vi "SP Perform Filter Bandwidth Limit Testing.vi"(6 "Limit Results In":T2={"Limit #"=0, "Parameter"={"Stimulus Port"=1, "Response Port"=0}, "Bandwidth Pass?"={"Pass?"=FALSE, "Bandwidth"=0.0, "Limit"=0.0, "Units"=enum."Hz"}, "Ripple Pass?"={"Pass?"=FALSE, "Ripple"=0.0, "Limit"=0.0, "Format"=enum."Log Mag"}, "Attenuation Results"=[], "Skirt Results"=[], "Pass?"=FALSE} {"Parameter"."Stimulus Port" min=1 step=1; "Parameter"."Response Port" min=1 step=1}, 8 "error in (no error)":errorcluster, 10 "Data":T10={"F0"=500.0, "dF"=1.0, "Formatted Values"=[-6.0, -6.0, -6.0, -6.0, -6.0, -6.0, -5.0, -4.0, -3.0, -2.0, -1.0017226002993769, -0.8636286738753696, -1.012432061728755, -0.8135188671805874, -1.084383696215112, -1.192695586219516, -0.8228939725524264, -1.1588169801015764, -1.0069715761898415, -0.8118111488159718, -0.9516999033989667, -1.0842662636672022, -1.0261931083967077, -0.816874162233468, -0.8335770068326294, -1.1794529347576463, -1.1032959879886735, -1.197742447623333, -0.9631229100196212, -0.9908453124177325, -0.9835470980893588, -1.10217991844936, -0.8956607286257672, -0.8794782872077156, -0.9013683651609963, -1.0772188731817596, -0.992723355191172, -0.9536275499498994, -0.9874327685983141, -0.921963653527827, -0.8848787728556787, -1.1874980208218, -0.996957511881206, -0.9972503730309241, -0.8866139538542095, -1.07344181331393, -0.881559772443858, -1.0112449407130875, -0.9865384477979471, -0.9901446738263366, -1.1718630063784758, -0.9951725256878827, -0.931778781153855, -0.9846289731021831, -0.851763264124267, -0.9086965469391421, -0.8349429101974368, -0.8383742350256687, -1.106571816484691, -0.9554005266395742, -0.9376822403043366, -1.131287512516927, -1.0382288806403288, -0.917054052988136, -0.9489467877812984, -0.9264227759143271, -1.0918690925892351, -1.1668737446636852, -1.0021735712381068, -1.1541225361979714, -1.1931131329605709, -0.8730502330378824, -0.850411285659811, -1.137775166801135, -1.1870586525662095, -1.0926571181161528, -1.118993526927924, -1.1211410787283602, -0.8920697041785735, -0.888430731015914, -1.0656600076605476, -1.1666787859795846, -1.0713340188424678, -0.8625910088884297, -1.1434360227216422, -0.9217710376784376, -1.1218396445954617, -0.9558195687190933, -1.1773692443654946, -1.0827782751424972, -1.1567791336122029, -0.8684407402614696, -0.8177845157195978, -0.9040657051180614, -0.9313557288389804, -1.0236831450620423, -1.050426714979035, -0.8344777069605718, -0.8274082929927138, -1.1990080831766776, -1.0947798998491134, -1.1963114865246718, -1.0016247375583676, -1.0877110100652403, -1.1556028882288836, -1.1918380581525247, -0.9751292214691399, -0.8884133044813358, -1.0347444321214612, -0.9445125246491541, -2.0, -3.0, -4.0, -5.0, -6.0, -6.0, -6.0, -6.0, -6.0, -6.0]}, 11 "Filter Limit":T11={"Limit #"=1, "Parameter"={"Stimulus Port"=1, "Response Port"=2}, "Format"=enum."Log Mag", "Filter Type"=enum."Bandpass", "Passband"={"Start/Center"=510.0, "Stop/Span"=610.0, "Units"=enum."MHz", "Freq Format"=enum."Start/Stop", "Bandwidth Attn"=3.0, "Passband Limit"=FALSE}, "Ripple"={"Ripple Limit"=TRUE, "Window On"=FALSE, "Ripple"=0.1, "Window"=10.0, "Units"=enum."MHz"}, "Attenuation Points"=[], "Skirt Points"=[]} {"Parameter"."Stimulus Port" min=1 step=1; "Parameter"."Response Port" min=1 step=1; "Passband"."Bandwidth Attn" format="%.3g"; "Passband"."Stop/Span" format="%.3g"; "Passband"."Start/Center" format="%.3g"}) -> (0 "error out":errorcluster, 2 "Results":T1, 3 "Pass?":bool, 4 "Limit Results Out":T2={"Limit #"=0, "Parameter"={"Stimulus Port"=1, "Response Port"=0}, "Bandwidth Pass?"={"Pass?"=FALSE, "Bandwidth"=0.0, "Limit"=0.0, "Units"=enum."Hz"}, "Ripple Pass?"={"Pass?"=FALSE, "Ripple"=0.0, "Limit"=0.0, "Format"=enum."Log Mag"}, "Attenuation Results"=[], "Skirt Results"=[], "Pass?"=FALSE} {"Parameter"."Stimulus Port" min=1 step=1; "Parameter"."Response Port" min=1 step=1})   [LabVIEW 2011]
uses:
  TypeDefs/SP Filter.ctl
  TypeDefs/SP Parameter.ctl
  TypeDefs/SP Format.ctl
  TypeDefs/SP Filter Type.ctl
  TypeDefs/SP Filter Passband.ctl
  TypeDefs/SP Frequency Units.ctl
  TypeDefs/SP Frequency Format.ctl
  TypeDefs/SP Filter Ripple.ctl
  TypeDefs/SP Attenuation Point.ctl
  TypeDefs/SP Attenuation Type.ctl
  TypeDefs/SP Skirt Rejection Point.ctl
  TypeDefs/SP Relative Loss.ctl
  TypeDefs/SP Limit Results.ctl
  TypeDefs/SP Bandwidth Limit Results.ctl
  TypeDefs/SP Ripple Limit Results.ctl
  TypeDefs/SP Attenuation Limit Results.ctl
  TypeDefs/SP Skirt Limit Results.ctl
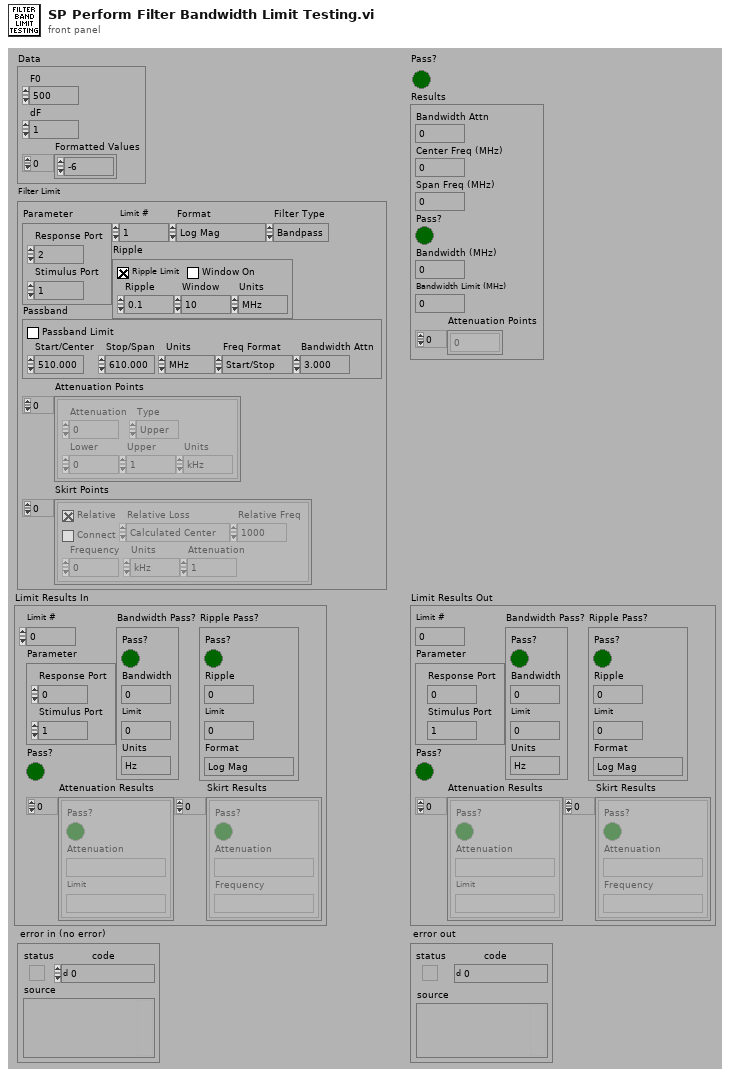
[diagram p1: front panel]
types:
  T1 = cluster{"Bandwidth Attn":dbl, "Center Freq (MHz)":dbl, "Span Freq (MHz)":dbl, "Pass?":bool, "Bandwidth (MHz)":dbl, "Bandwidth Limit (MHz)":dbl, "Attenuation Points":dbl[]}
  T2 = typedef "SP Limit Results.ctl" = cluster{"Limit #":i8, "Parameter":T3, "Bandwidth Pass?":T4, "Ripple Pass?":T6, "Attenuation Results":T8[], "Skirt Results":T9[], "Pass?":bool}
  T3 = typedef "SP Parameter.ctl" = cluster{"Stimulus Port":i8, "Response Port":i8}
  T4 = typedef "SP Bandwidth Limit Results.ctl" = cluster{"Pass?":bool, "Bandwidth":dbl, "Limit":dbl, "Units":T5}
  T5 = typedef "SP Frequency Units.ctl" = enum16{"Hz", "kHz", "MHz", "GHz", "Points"}
  T6 = typedef "SP Ripple Limit Results.ctl" = cluster{"Pass?":bool, "Ripple":dbl, "Limit":dbl, "Format":T7}
  T7 = typedef "SP Format.ctl" = enum16{"Log Mag", "Lin Mag", "SWR", "Phase", "Expanded Phase", "Delay", "Insertion Loss", "Isolation", "Return Loss"}
  T8 = typedef "SP Attenuation Limit Results.ctl" = cluster{"Pass?":bool, "Attenuation":string, "Limit":string}
  T9 = typedef "SP Skirt Limit Results.ctl" = cluster{"Pass?":bool, "Attenuation":string, "Frequency":string}
  T10 = cluster{"F0":dbl, "dF":dbl, "Formatted Values":dbl[]}
  T11 = typedef "SP Filter.ctl" = cluster{"Limit #":i8, "Parameter":T3, "Format":T7, "Filter Type":T12, "Passband":T13, "Ripple":T15, "Attenuation Points":T16[], "Skirt Points":T18[]}
  T12 = typedef "SP Filter Type.ctl" = enum16{"Lowpass", "Highpass", "Bandpass", "Bandstop"}
  T13 = typedef "SP Filter Passband.ctl" = cluster{"Start/Center":dbl, "Stop/Span":dbl, "Units":T5, "Freq Format":T14, "Bandwidth Attn":dbl, "Passband Limit":bool}
  T14 = typedef "SP Frequency Format.ctl" = enum16{"Start/Stop", "Center/Span"}
  T15 = typedef "SP Filter Ripple.ctl" = cluster{"Ripple Limit":bool, "Window On":bool, "Ripple":dbl, "Window":dbl, "Units":T5}
  T16 = typedef "SP Attenuation Point.ctl" = cluster{"Attenuation":dbl, "Type":T17, "Lower":dbl, "Upper":dbl, "Units":T5}
  T17 = typedef "SP Attenuation Type.ctl" = enum16{"Center", "Lower", "Upper"}
  T18 = typedef "SP Skirt Rejection Point.ctl" = cluster{"Relative":bool, "Connect":bool, "Frequency":dbl, "Units":T5, "Attenuation":dbl, "Relative Loss":T19, "Relative Freq":dbl}
  T19 = typedef "SP Relative Loss.ctl" = enum16{"Calculated Center", "Passband Minimum", "Passband Maximum", "Passband Average", "Frequency"}
  T20 = cluster{"Bandwidth Attn":dbl, "Start/Center Out":dbl, "Stop/Span Out":dbl, bool, "Interpolated X Value":dbl, "Stop/Span Out":dbl, dbl[]}
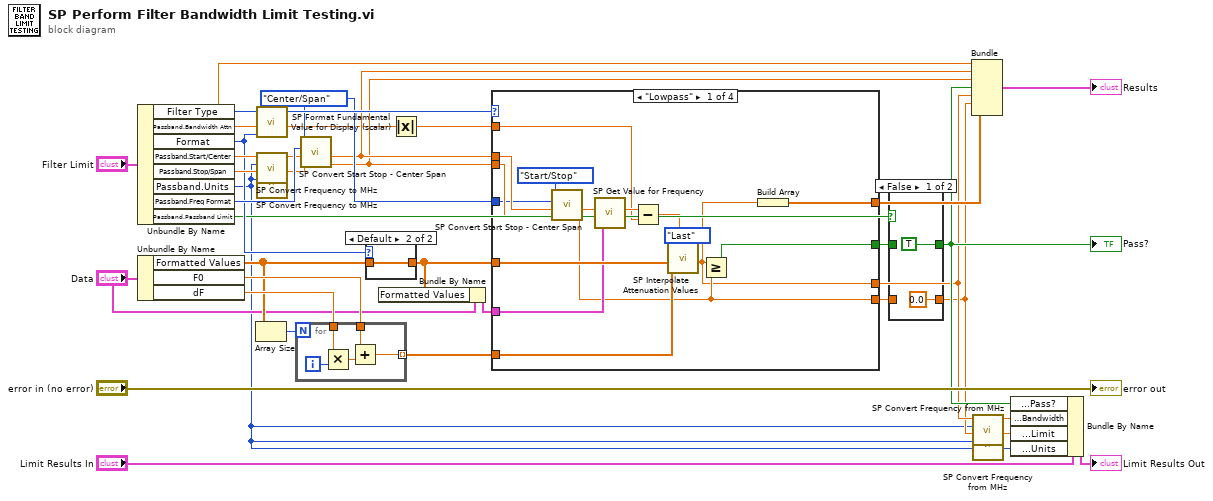
[diagram p0: block diagram]
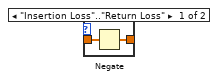
[diagram p3: hidden frame]
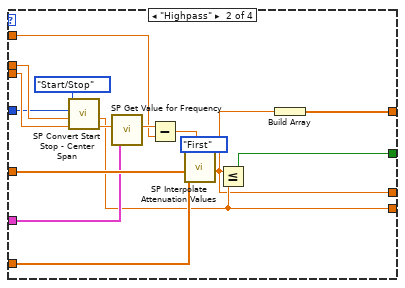
[diagram p4: hidden frame]
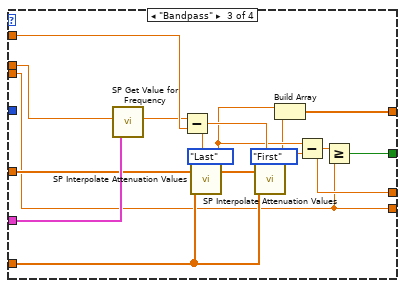
[diagram p5: hidden frame]
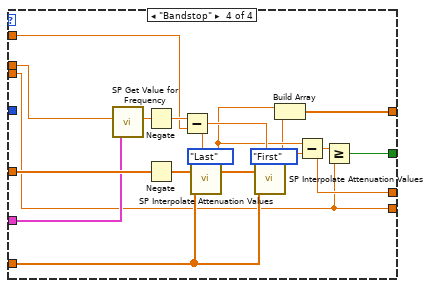
[diagram p6: hidden frame]
diagram:
  w17 = SP_Frequency_Format."Center/Span" ("Freq Format To")
  n1 = Unbundle By Name("Filter Limit") -> ("Filter Type"=w35:T12, "Passband.Bandwidth Attn"=w25:dbl, "Format"=w24:T7, "Passband.Start/Center"=w34:dbl, "Passband.Stop/Span"=w33:dbl, "Passband.Units"=w1:T5, "Passband.Freq Format"=w27:T14, "Passband.Passband Limit"=w9:bool)
  n2 = Unbundle By Name("Data") -> ("Formatted Values"=w23:dbl[], "F0"=w32:dbl, "dF"=w31:dbl)
  n3 = Array Size(array=w23) -> (size(s)=w21:i32)
  n4 = call "SP Format Fundamental Value for Display (scalar).vi"("Format"=w24, "Stored Value (0, linear)"=w25) -> ("Display Value"=w14:dbl)  [unwired: 5 out]
  n5 = call "SP Convert Frequency to MHz.vi"("Units"=w1, "Frequency"=w34) -> ("Converted Frequency"=w19:dbl)  [unwired: 1 in, 8 out]
  n6 = call "SP Convert Frequency to MHz.vi"("Units"=w1, "Frequency"=w33) -> ("Converted Frequency"=w18:dbl)  [unwired: 1 in, 8 out]
  n7 = for {
    N: w21 -> [_]
    tunnel: w31 -> [w40]
    tunnel: w32 -> [w38]
    tunnel: [w37] -> w20 mode=indexing
    i -> [w41]
    n8 = Multiply(x=w40, y=w41) -> (x*y=w39:dbl)
    n9 = Add(x=w38, y=w39) -> (x+y=w37:dbl)
  }
  n10 = call "SP Convert Start Stop - Center Span.vi"("Stop/Span In"=w18, "Start/Center In"=w19, "Freq Format From"=w27, "Freq Format To"=w17) -> ("Stop/Span Out"=w15:dbl, "Start/Center Out"=w16:dbl)  [unwired: 6 out]
  n11 = case shown="Default" w24 {
    tunnel: w23 -> [w43 w44]
    tunnel: [w42 w44] -> w11
    frame "Insertion Loss".."Return Loss" {
      n12 = Negate(x=w43) -> (-x=w42:dbl[])
    }
    frame Default {
    }
  }
  n13 = Bundle By Name(cluster="Data", "Formatted Values"=w11) -> (w12:T10)
  n14 = Absolute Value(x=w14) -> (abs(x)=w13:dbl)
  n15 = case shown="\"Lowpass\"" w35 {
    tunnel: w16 -> [w56 w72 w81 w95]
    tunnel: w15 -> [w55 w71 w80 w96]
    tunnel: w17 -> [w54 w70 _ _]
    tunnel: w11 -> [w59 w75 w84 w102]
    tunnel: w13 -> [w51 w67 w86 w99]
    tunnel: w20 -> [w58 w74 w88 w101]
    tunnel: w12 -> [w53 w69 w87 w100]
    tunnel: [w49 w65 w85 w98] -> w8
    tunnel: [w46 w61 w82 w97] -> w5
    tunnel: [w47 w63 w80 w96] -> w7
    tunnel: [w45 w62 w77 w92] -> w10
    frame "Lowpass" {
      n16 = call "SP Convert Start Stop - Center Span.vi"("Stop/Span In"=w55, "Start/Center In"=w56, "Freq Format From"=w54, "Freq Format To"=SP_Frequency_Format."Start/Stop") -> ("Stop/Span Out"=w47:dbl, "Start/Center Out"=w48:dbl)  [unwired: 6 out]
      n17 = call "SP Get Value for Frequency.vi"("Data"=w53, "Frequency (MHz)"=w48) -> ("Value"=w52:dbl)  [unwired: 5 out]
      n18 = Subtract(x=w52, y=w51) -> (x-y=w50:dbl)
      n19 = call "SP Interpolate Attenuation Values.vi"("Instance (First)"=enum16{"First", "Last"}."Last", "Attenuation Value"=w50, "X Values"=w58, "Y Values"=w59) -> ("Interpolated X Value"=w46:dbl)  [unwired: 7 out]
      n20 = Greater Or Equal?(x=w46, y=w47) -> (x >= y?=w49:bool)
      n21 = Build Array(w46) -> (w45:dbl[])
    }
    frame "Highpass" {
      n22 = call "SP Convert Start Stop - Center Span.vi"("Stop/Span In"=w71, "Start/Center In"=w72, "Freq Format From"=w70, "Freq Format To"=SP_Frequency_Format."Start/Stop") -> ("Stop/Span Out"=w64:dbl, "Start/Center Out"=w63:dbl)  [unwired: 6 out]
      n23 = call "SP Get Value for Frequency.vi"("Data"=w69, "Frequency (MHz)"=w64) -> ("Value"=w68:dbl)  [unwired: 5 out]
      n24 = Subtract(x=w68, y=w67) -> (x-y=w66:dbl)
      n25 = call "SP Interpolate Attenuation Values.vi"("Instance (First)"=enum16{"First", "Last"}."First", "Attenuation Value"=w66, "X Values"=w74, "Y Values"=w75) -> ("Interpolated X Value"=w61:dbl)  [unwired: 7 out]
      n26 = Less Or Equal?(x=w61, y=w63) -> (x <= y?=w65:bool)
      n27 = Build Array(w61) -> (w62:dbl[])
    }
    frame "Bandpass" {
      n28 = call "SP Get Value for Frequency.vi"("Data"=w87, "Frequency (MHz)"=w81) -> ("Value"=w83:dbl)  [unwired: 5 out]
      n29 = Subtract(x=w83, y=w86) -> (x-y=w89:dbl)
      n30 = call "SP Interpolate Attenuation Values.vi"("Instance (First)"=enum16{"First", "Last"}."Last", "Attenuation Value"=w89, "X Values"=w88, "Y Values"=w84) -> ("Interpolated X Value"=w79:dbl)  [unwired: 7 out]
      n31 = call "SP Interpolate Attenuation Values.vi"("Instance (First)"=enum16{"First", "Last"}."First", "Attenuation Value"=w89, "X Values"=w88, "Y Values"=w84) -> ("Interpolated X Value"=w78:dbl)  [unwired: 7 out]
      n32 = Build Array(w79, w78) -> (w77:dbl[])
      n33 = Subtract(x=w79, y=w78) -> (x-y=w82:dbl)
      n34 = Greater Or Equal?(x=w82, y=w80) -> (x >= y?=w85:bool)
    }
    frame "Bandstop" {
      n35 = call "SP Get Value for Frequency.vi"("Data"=w100, "Frequency (MHz)"=w95) -> ("Value"=w105:dbl)  [unwired: 5 out]
      n36 = Negate(x=w105) -> (-x=w103:dbl)
      n37 = Negate(x=w102) -> (-x=w104:dbl[])
      n38 = Subtract(x=w103, y=w99) -> (x-y=w106:dbl)
      n39 = call "SP Interpolate Attenuation Values.vi"("Instance (First)"=enum16{"First", "Last"}."Last", "Attenuation Value"=w106, "X Values"=w101, "Y Values"=w104) -> ("Interpolated X Value"=w94:dbl)  [unwired: 7 out]
      n40 = call "SP Interpolate Attenuation Values.vi"("Instance (First)"=enum16{"First", "Last"}."First", "Attenuation Value"=w106, "X Values"=w101, "Y Values"=w104) -> ("Interpolated X Value"=w93:dbl)  [unwired: 7 out]
      n41 = Build Array(w94, w93) -> (w92:dbl[])
      n42 = Subtract(x=w94, y=w93) -> (x-y=w97:dbl)
      n43 = Greater Or Equal?(x=w97, y=w96) -> (x >= y?=w98:bool)
    }
  }
  n44 = case shown="False" w9 {
    tunnel: w8 -> [_ w111]
    tunnel: w7 -> [_ w112]
    tunnel: [0.0 ("Stop/Span Out") w112] -> w4
    tunnel: [TRUE w111] -> w6
    frame False {
    }
    frame True {
    }
  }
  "Pass?" <- w6
  n45 = Bundle("Bandwidth Attn"=w25, "Start/Center Out"=w16, "Stop/Span Out"=w15, w6, "Interpolated X Value"=w5, "Stop/Span Out"=w4, w10) -> (→"Results":T20)  [unwired: 1 out]
  n46 = call "SP Convert Frequency from MHz.vi"("Units"=w1, "Frequency (MHz)"=w5) -> ("Converted Frequency"=w2:dbl)  [unwired: 1 in, 8 out]
  n47 = call "SP Convert Frequency from MHz.vi"("Units"=w1, "Frequency (MHz)"=w4) -> ("Converted Frequency"=w3:dbl)  [unwired: 1 in, 8 out]
  n48 = Bundle By Name(cluster="Limit Results In", "Bandwidth Pass?.Pass?"=w6, "Bandwidth Pass?.Bandwidth"=w2, "Bandwidth Pass?.Limit"=w3, "Bandwidth Pass?.Units"=w1) -> (→"Limit Results Out":T2)
  "error out" <- "error in (no error)"
